vi "New.vi"(11 "VISA resource name":refnum<visa-resource-name>) -> (0 "error out":errorcluster, 3 "Motor_Serial out":refnum<class "Serial.lvclass">)   [LabVIEW 2019, in "Serial.lvclass"]
uses:
  Serial.lvclass
  <vilib>/Instr/_visa.llb/VISA Flush IO Buffer Mask.ctl
  Serial.lvclass/Serial.ctl
panel:
  in  "Mask":T1=16 items=["Flush Receive Buffer"=16, "Write Transmit Buffer to Device"=32, "Flush Receive Buffer (No I/O)"=64, "Flush Transmit Buffer"=128]
  in  "Message Based Settings:Suppress End Enable":bool
  in  "Message Based Settings:Send End Enable":bool
  in  "Message Based Settings:Termination Character Enable":bool
  in  "Serial Settings:End Mode for Writes":u16(ring)=2 items=["None", "Last Bit", "TermChar", "Break"]
  in  "Serial Settings:End Mode for Reads":u16(ring)=2 items=["None", "Last Bit", "TermChar"]
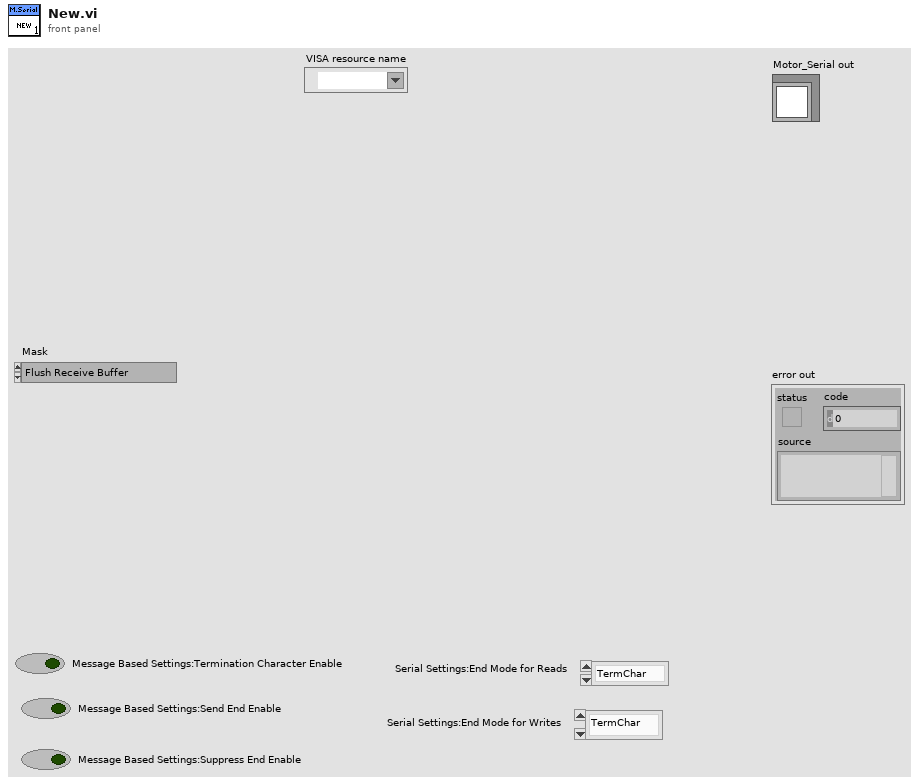
[diagram p1: front panel]
types:
  T1 = typedef "VISA Flush IO Buffer Mask.ctl" = u16
  T2 = typedef "Semaphore RefNum" = refnum<k1>
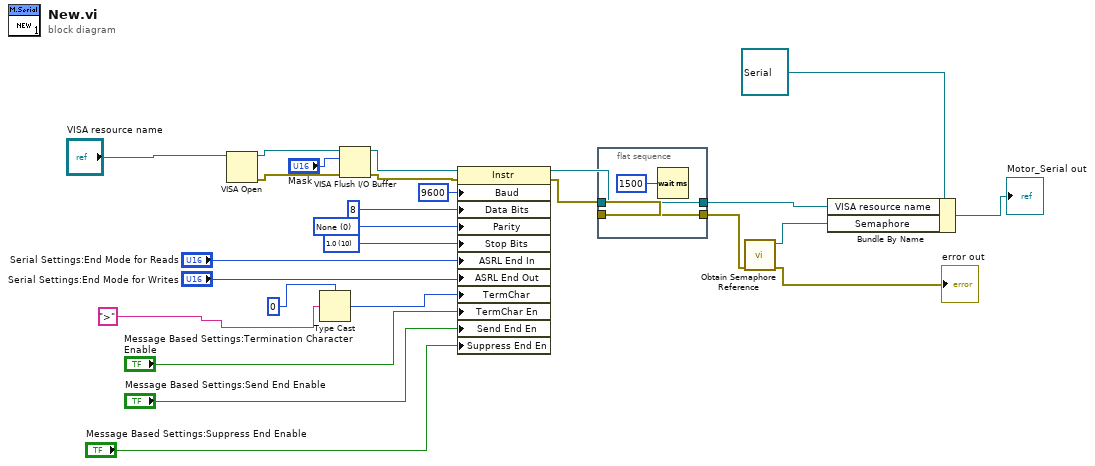
[diagram p0: block diagram]
diagram:
  w24 = u16 10 items=["1.0"=10, "1.5"=15, "2.0"=20] ("Serial Settings:Stop Bits")
  w25 = u16 0 items=["None", "Odd", "Even", "Mark", "Space"] ("Serial Settings:Parity")
  n1 = VISA Open(VISA resource name="VISA resource name") -> (VISA resource name=w15:refnum<visa-resource-name>, error out=w12:errorcluster)  [unwired: 4 in]
  n2 = Type Cast(type=u8 0, x=">") -> (*(type *) &x=w20:u8)
  n3 = VISA Flush I/O Buffer(VISA resource name=w15, mask (16)="Mask", error in (no error)=w12) -> (VISA resource name out=w14:refnum<visa-resource-name>, error out=w13:errorcluster)
  n4 = property class="Instr"(reference=w14, error in=w13, "Baud"=u32 9600 ("Serial Settings:Baud Rate"), "Data Bits"=u16 8 ("Serial Settings:Data Bits"), "Parity"=w25, "Stop Bits"=w24, "ASRL End In"="Serial Settings:End Mode for Reads", "ASRL End Out"="Serial Settings:End Mode for Writes", "TermChar"=w20, "TermChar En"="Message Based Settings:Termination Character Enable", "Send End En"="Message Based Settings:Send End Enable", "Suppress End En"="Message Based Settings:Suppress End Enable") -> (reference out=w9:refnum<visa-resource-name>, error out=w10:errorcluster)
  n5 = flat-sequence {
    tunnel: [w28] -> w6
    tunnel: w9 -> [w28]
    tunnel: w10 -> [w27]
    tunnel: [w27] -> w4
    frame #0 {
      n6 = Wait (ms)(milliseconds to wait=u32 1500) -> ()  [unwired: 1 out]
    }
  }
  n7 = call <vilib>:"Obtain Semaphore Reference.vi"("error in (no error)"=w4) -> ("error out"=→"error out":errorcluster, "semaphore"=w2:T2)  [unwired: 4 in, 1 out]
  n8 = Bundle By Name(cluster=refnum<class "Serial.lvclass"> refnum ("Motor_Serial.lvclass"), "VISA resource name"=w6, "Semaphore"=w2) -> (→"Motor_Serial out":refnum<class "Serial.lvclass">)
